vi "Main.vi"(0 "Data":dbl, 5 "Stop":bool, 11 "Error in":errorcluster) -> (4 "Data Out":dbl, 15 "Error out":errorcluster)   [LabVIEW 2020, in "DVR Access.lvlib"]
uses:
  DVR Access.lvlib
  Typedefs/Data Cluster.ctl
  Typedefs/LV2 Operations.ctl
  DVR Handson.lvlib
panel:
  # "This system is used to get data \nfrom DVR ref and manipulate it\nin multiple loops and finally find\nthe outcomes"
  # "DVR ACCESS"
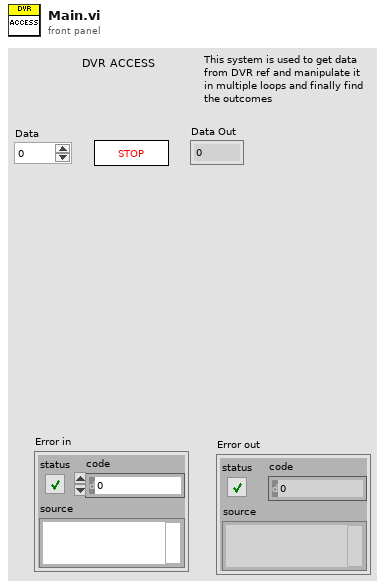
[diagram p1: front panel]
types:
  T1 = typedef "DVR Handson.lvlib/LV2 Operations.ctl" = enum16{"Initialize", "Read", "Write"}
  T2 = typedef "DVR Access.lvlib/Data Cluster.ctl" = cluster{"Data":dbl, "Stop":bool}
  T3 = typedef "Data Cluster.ctl" = cluster{"Data":dbl, "Stop":bool}
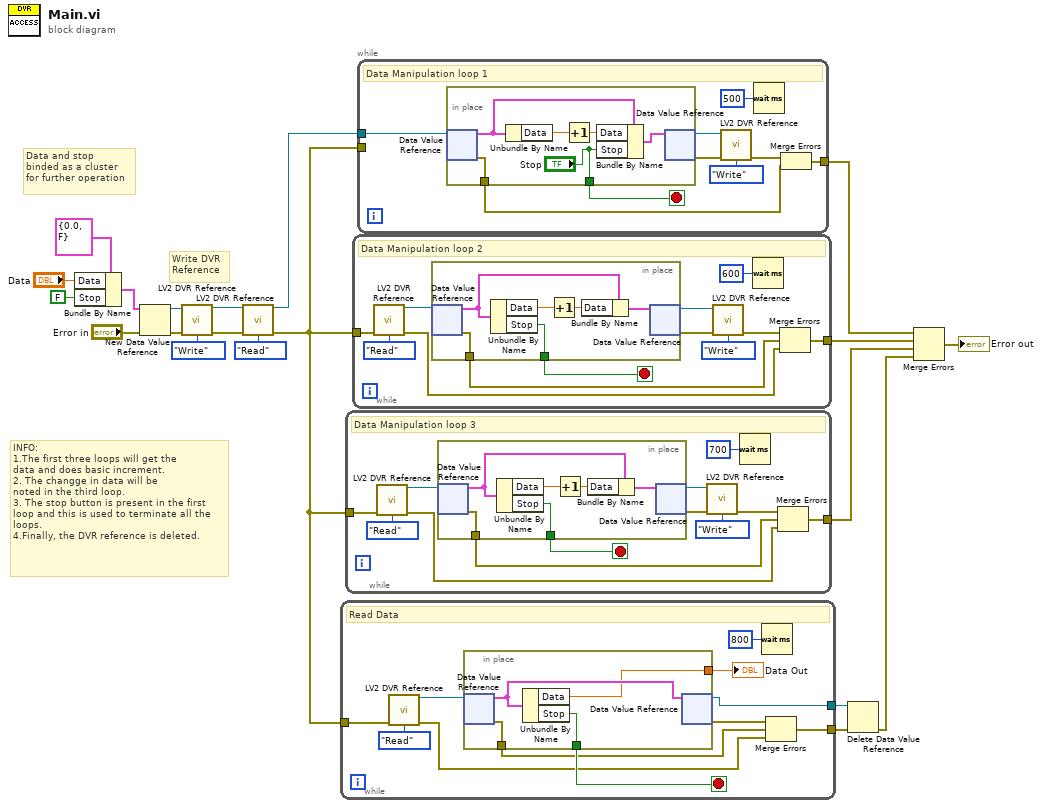
[diagram p0: block diagram]
diagram:
  # "INFO:\n1.The first three loops will get the\ndata and does basic increment.\n2. The changge in data will be \nnoted in the third loop.\n3. The stop button is present in the first \nloop and this is used to terminate all the \nloops.\n4.Finally, the DVR reference is deleted."
  # "Write DVR \nReference"
  # "Data and stop\nbinded as a cluster \nfor further operation"
  n1 = Bundle By Name(cluster=T2 {"Data"=0.0, "Stop"=FALSE}, "Data"="Data", "Stop"=FALSE) -> (w17:T2)
  n2 = New Data Value Reference(data value=w17, error in="Error in") -> (data value reference=w14:refnum<data-value>, error out=w16:errorcluster)
  n3 = call "LV2 DVR Reference.vi"("DVR Input"=w14, "Error in"=w16, "Operation"=LV2_Operations."Write") -> ("DVR Output"=w8:refnum<data-value>, "Error out"=w7:errorcluster)  [unwired: 11 in]
  n4 = call "LV2 DVR Reference.vi"("DVR Input"=w8, "Error in"=w7, "Operation"=LV2_Operations."Read") -> ("DVR Output"=w4:refnum<data-value>, "Error out"=w6:errorcluster)  [unwired: 11 in]
  n5 = while {
    tunnel: w6 -> [w24]
    tunnel: [w26] -> w3
    tunnel: [w21] -> w2
    stop <- w30 stop-if-true
    # "Read Data"
    n6 = call "LV2 DVR Reference.vi"("Error in"=w24, "Operation"=LV2_Operations."Read") -> ("DVR Output"=w23:refnum<data-value>, "Error out"=w22:errorcluster)  [unwired: 12 in]
    n7 = in-place {
      in-place-border: [w35] -> w30
      in-place-border: [w34] -> w28
      in-place-border: [w32] -> w31
      n8 = in-place-dvr #1(w23) -> (w33:T3, w34:errorcluster)
      n9 = Unbundle By Name(w33) -> ("Data"=w32:dbl, "Stop"=w35:bool)
      n10 = in-place-dvr #1(w33) -> (w21:refnum<data-value>, w29:errorcluster)
    }
    "Data Out" <- w31
    n11 = Wait (ms)(milliseconds to wait=u32 800) -> ()  [unwired: 1 out]
    n12 = Merge Errors(w29, w28, w22) -> (w26:errorcluster)
  }
  n13 = while {
    tunnel: w6 -> [w38]
    tunnel: [w41] -> w11
    stop <- w47 stop-if-true
    # "Data Manipulation loop 3"
    n14 = call "LV2 DVR Reference.vi"("Error in"=w38, "Operation"=LV2_Operations."Read") -> ("DVR Output"=w37:refnum<data-value>, "Error out"=w36:errorcluster)  [unwired: 12 in]
    n15 = in-place {
      in-place-border: [w49] -> w47
      in-place-border: [w48] -> w42
      n16 = in-place-dvr #2(w37) -> (w51:T3, w48:errorcluster)
      n17 = Unbundle By Name(w51) -> ("Data"=w53:dbl, "Stop"=w49:bool)
      n18 = Increment(x=w53) -> (x+1=w52:dbl)
      n19 = Bundle By Name(cluster=w51, "Data"=w52) -> (w50:T3)
      n20 = in-place-dvr #2(w50) -> (w45:refnum<data-value>, w44:errorcluster)
    }
    n21 = call "LV2 DVR Reference.vi"("DVR Input"=w45, "Error in"=w44, "Operation"=LV2_Operations."Write") -> ("Error out"=w43:errorcluster)  [unwired: 11 in, 1 out]
    n22 = Wait (ms)(milliseconds to wait=u32 700) -> ()  [unwired: 1 out]
    n23 = Merge Errors(w43, w42, w36) -> (w41:errorcluster)
  }
  n24 = while {
    tunnel: w6 -> [w56]
    tunnel: [w59] -> w10
    stop <- w65 stop-if-true
    # "Data Manipulation loop 2"
    n25 = call "LV2 DVR Reference.vi"("Error in"=w56, "Operation"=LV2_Operations."Read") -> ("DVR Output"=w55:refnum<data-value>, "Error out"=w54:errorcluster)  [unwired: 12 in]
    n26 = in-place {
      in-place-border: [w67] -> w65
      in-place-border: [w66] -> w60
      n27 = in-place-dvr #3(w55) -> (w69:T3, w66:errorcluster)
      n28 = Unbundle By Name(w69) -> ("Data"=w71:dbl, "Stop"=w67:bool)
      n29 = Increment(x=w71) -> (x+1=w70:dbl)
      n30 = Bundle By Name(cluster=w69, "Data"=w70) -> (w68:T3)
      n31 = in-place-dvr #3(w68) -> (w62:refnum<data-value>, w63:errorcluster)
    }
    n32 = call "LV2 DVR Reference.vi"("DVR Input"=w62, "Error in"=w63, "Operation"=LV2_Operations."Write") -> ("Error out"=w61:errorcluster)  [unwired: 11 in, 1 out]
    n33 = Wait (ms)(milliseconds to wait=u32 600) -> ()  [unwired: 1 out]
    n34 = Merge Errors(w61, w60, w54) -> (w59:errorcluster)
  }
  n35 = while {
    tunnel: w6 -> [_]
    tunnel: [w78] -> w9
    tunnel: w4 -> [w72]
    stop <- w80 stop-if-true
    # "Data Manipulation loop 1"
    n36 = in-place {
      in-place-border: ["Stop"] -> w80
      in-place-border: [w81] -> w79
      n37 = in-place-dvr #4(w72) -> (w84:T3, w81:errorcluster)
      n38 = Unbundle By Name(w84) -> ("Data"=w86:dbl)
      n39 = Increment(x=w86) -> (x+1=w85:dbl)
      n40 = Bundle By Name(cluster=w84, "Data"=w85, "Stop"="Stop") -> (w82:T3)
      n41 = in-place-dvr #4(w82) -> (w73:refnum<data-value>, w75:errorcluster)
    }
    n42 = call "LV2 DVR Reference.vi"("DVR Input"=w73, "Error in"=w75, "Operation"=LV2_Operations."Write") -> ("Error out"=w74:errorcluster)  [unwired: 11 in, 1 out]
    n43 = Wait (ms)(milliseconds to wait=u32 500) -> ()  [unwired: 1 out]
    n44 = Merge Errors(w74, w79) -> (w78:errorcluster)
  }
  n45 = Delete Data Value Reference(data value reference=w2, error in=w3) -> (error out=w1:errorcluster)  [unwired: 1 out]
  n46 = Merge Errors(w9, w10, w11, w1) -> (→"Error out":errorcluster)
